vi "NavX Variable Get.vi"(8 "error in":errorcluster) -> ()   [LabVIEW 2018]
uses:
  <vilib>/Rock Robotics/SystemInterfaces/spilib/spi_bus.ctl
  navx-mxp/labview/navX Library v2/IO/Open/Z900_navX_Open_SPI.vi
  navx-mxp/labview/navX Library v2/navX Library v2.lvlib
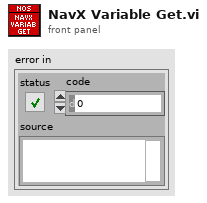
[diagram p1: front panel]
types:
  T1 = typedef "spi_bus.ctl" = enum16{"SPI On-Board, CS0", "SPI On-Board, CS1", "SPI On-Board, CS2", "SPI On-Board, CS3", "SPI MXP", "Invalid"}
  T2 = typedef "navX Library v2.lvlib/Z900_navX_DeviceTypeDef.ctl" = cluster{"Interface":cluster{"Protocol":T3, "Update Rate (4Hz-100Hz)":u8, "navX Open TypeDef":variant}, "Notify Packet":refnum<notifier>, "Loop VI Refnum":refnum<vi>, "Ready to Close Occurrence Refnum":refnum<k4>}
  T3 = typedef "navX Library v2.lvlib/Z900_navX_ProtocolTypeDef.ctl" = enum16{"SERIAL", "I2C", "SPI"}
  T4 = cluster{"Yaw":dbl, "Roll":dbl, "Pitch":dbl, "Heading":dbl, "Fused Heading":dbl}
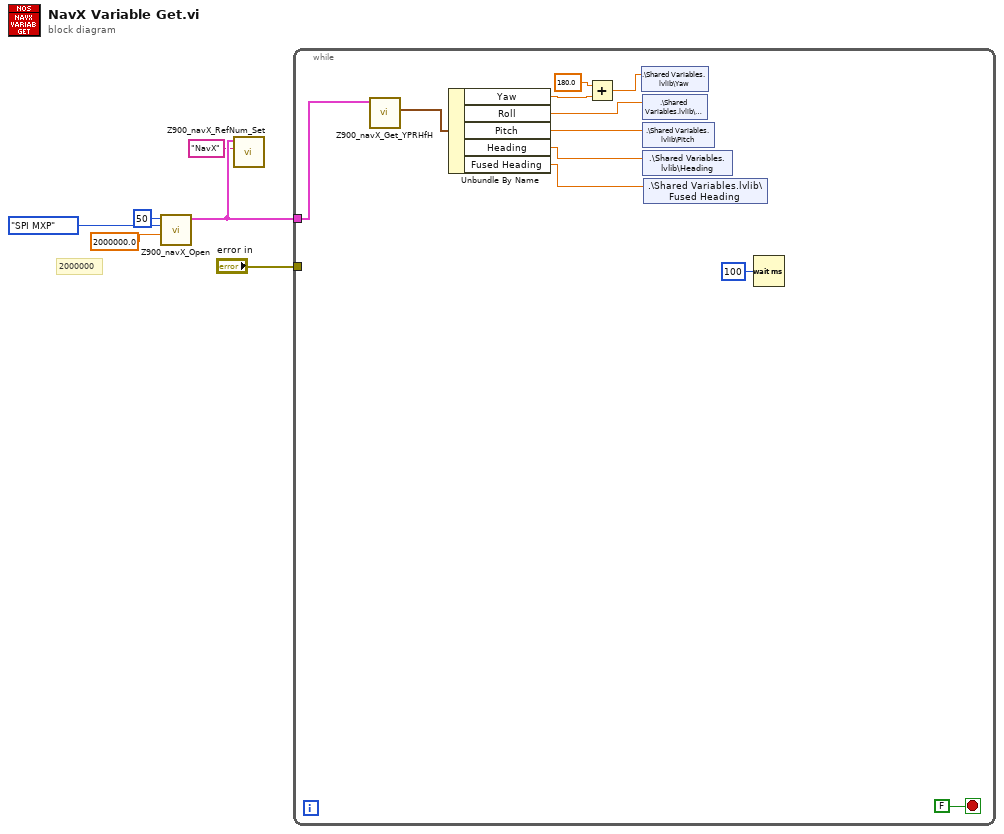
[diagram p0: block diagram]
diagram:
  # "2000000"
  n1 = call-poly "Z900_navX_Open.vi"("Clock Rate (Hz)"=2000000.0, "SPI Bus"=spi_bus."SPI MXP", "Update Rate (4Hz-60Hz)"=u8 50) -> ("navX Device"=w2:T2)  [unwired: 7 in, 1 out]
  n2 = call "Z900_navX_RefNum_Set.vi"("refnum name"="NavX", "navX Device"=w2) -> ()  [unwired: 8 in, 2 out]
  n3 = while {
    tunnel: "error in" -> [_]
    tunnel: w2 -> [w7]
    stop <- FALSE stop-if-true
    n4 = call "Z900_navX_Get_YPRHfH.vi"("navX Device"=w7) -> ("YRPHfH"=w8:T4)  [unwired: 7 in, 3 out]
    n5 = Unbundle By Name(w8) -> ("Yaw"=w13:dbl, "Roll"=w10:dbl, "Pitch"=w17:dbl, "Heading"=w16:dbl, "Fused Heading"=w15:dbl)
    n6 = Add(x=180.0, y=w13) -> (x+y=w9:dbl)
    n7 = shared-variable ".\\Shared Variables.lvlib\\Yaw"(w9) -> ()  [unwired: 1 in, 1 out]
    n8 = shared-variable ".\\Shared Variables.lvlib\\Roll"(w10) -> ()  [unwired: 1 in, 1 out]
    n9 = shared-variable ".\\Shared Variables.lvlib\\Pitch"(w17) -> ()  [unwired: 1 in, 1 out]
    n10 = shared-variable ".\\Shared Variables.lvlib\\Heading"(w16) -> ()  [unwired: 1 in, 1 out]
    n11 = shared-variable ".\\Shared Variables.lvlib\\Fused Heading"(w15) -> ()  [unwired: 1 in, 1 out]
    n12 = Wait (ms)(milliseconds to wait=u32 100) -> ()  [unwired: 1 out]
  }
